vi "FPGA Resampling (60 Hz).vi"(0 "signal in":fxp<+/-,24,1>, 1 "number of channels":T3=7 items=["1"=1, "2"=2, "3"=3, "4"=4, "5"=5, "6"=6, "7"=7, "8"=8, "9"=9, "10"=10, "11"=11, "12"=12, "13"=13, "14"=14, "15"=15, "16"=16, "17"=17, "18"=18, "19"=19, "20"=20, "21"=21, "22"=22, "23"=23, "24"=24, "25"=25, "26"=26, "27"=27, "28"=28, "29"=29, "30"=30, "31"=31, "32"=32], 5 "timestamp [s]":fxp<+,64,32> format="%.42g", 7 "reference channel index (0)":u8, 9 "input valid? (T)":bool=TRUE, 12 "ready for output? (T)":bool=TRUE, 13 "samples per cycle (192)":u16=192) -> (4 "resampled data":T2, 6 "resampling info":T1={"nominal frequency"=enum."50 Hz", "resampling valid?"=FALSE, "samples per cycle"=192}, 10 "output valid?":bool, 15 "error":i32)   [LabVIEW 2014, in "NI_EP_Resample_FPGA.lvlib"]
doc: "Resamples even-time-spaced voltage and current signals into even-angle-spaced signals. The input signals must have a sample rate of 50 kHz. The output signals are synchronous with the line frequency with a constant number of samples per cycle. Use the Resampling for Power Quality VI if you want to perform resampling on the host computer. You must manually select the polymorphic instance to use.\n\nThis VI supports measuring single-bus single-line and single-bus multiple-line systems."
uses:
  <vilib>/addons/Electrical Power/PQ/Resampling/NI_EP_Resample_FPGA.lvlib
  <vilib>/addons/Electrical Power/PQ/Resampling/FPGA/subVIs/fpga_Typedef Fnom.ctl
  <vilib>/addons/Electrical Power/PQ/Resampling/FPGA/subVIs/fpga_Resampling Info.ctl
  <vilib>/addons/Electrical Power/PQ/Resampling/FPGA/subVIs/fpga_Resampled.ctl
  <vilib>/addons/Electrical Power/PQ/Resampling/FPGA/subVIs/fpga_NofCH (32ch).ctl
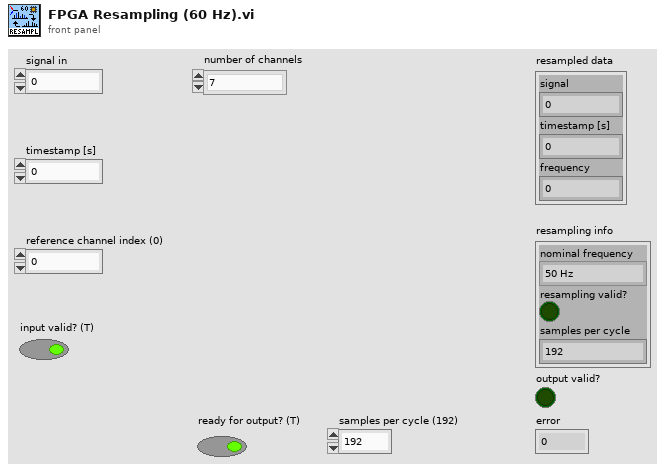
[diagram p1: front panel]
types:
  T1 = typedef "NI_EP_Resample_FPGA.lvlib/fpga_Resampling Info.ctl" = cluster{"nominal frequency":enum16{"50 Hz", "60 Hz"}, "resampling valid?":bool, "samples per cycle":u16}
  T2 = typedef "NI_EP_Resample_FPGA.lvlib/fpga_Resampled.ctl" = cluster{"signal":fxp<+/-,32,3>, "timestamp [s]":fxp<+,64,32>, "frequency":fxp<+,32,8>}
  T3 = typedef "NI_EP_Resample_FPGA.lvlib/fpga_NofCH (32ch).ctl" = u8
  T4 = typedef "NI_EP_Resample_FPGA.lvlib/fpga_Typedef Fnom.ctl" = u8
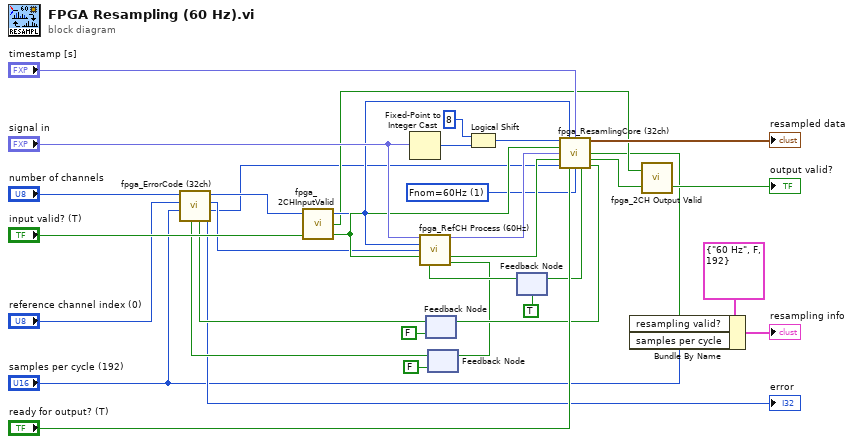
[diagram p0: block diagram]
diagram:
  w14 = T4 1 items=["Fnom=50Hz", "Fnom=60Hz"] ("Fnom")
  n1 = Fixed-Point to Integer Cast(1:"signal in") -> (0:w22:i32)
  n2 = feedback #1(FALSE) -> (w5:bool)
  n3 = feedback #2(FALSE) -> (w6:bool)
  n4 = call <vilib>:"fpga_ErrorCode (32ch).vi"("resampling FIFO time in"=w5, "Ref filter FIFO time in"=w6, "samples per cycle"="samples per cycle (192)", "reference channel index"="reference channel index (0)", "number of channels"="number of channels") -> ("error"=→"error":i32, "samples per cycle out"=w11:u16, "ref channel index out"=w12:u8, "number of CH out"=w13:u8)  [unwired: 3 in]
  n5 = call <vilib>:"fpga_2CHInputValid.vi"("input data valid"="input valid? (T)", "Channel number"=w13) -> ("input valid"=w24:bool, "1CH?"=w16:bool, "Channel number"=w17:u8)  [unwired: 1 in]
  n6 = Logical Shift(y=i8 8, x=w22) -> (x << y=w20:i32)
  n7 = feedback #3(TRUE ("Ready for reference input")) -> (w23:bool)
  n8 = call <vilib>:"fpga_RefCH Process (60Hz).vi"("data in <?24.1>"="signal in", "Channel number"=w17, "Reference index"=w12, "input data valid"=w24, "ready for output"=w23) -> ("Filtered Ref data <24,3>"=w19:fxp<+/-,24,3>, "output valid"=w18:bool, "Timed Out"=w7:bool)  [unwired: 8 in]
  n9 = feedback-in #2(w7) -> ()
  n10 = call <vilib>:"fpga_ResamlingCore (32ch).vi"("data in"=w20, "Channel number"=w17, "timestamp"="timestamp [s]", "input data valid"=w24, "reference in"=w19, "input reference valid"=w18, "interpolation factor"=w11, "Ready for output"="ready for output? (T)", "Fnom"=w14) -> ("Resample data and time"=→"resampled data":T2, "resampling valid"=w3:bool, "output valid"=w15:bool, "Ready for reference input"=w26:bool, "FIFO timeout?"=w9:bool)  [unwired: 2 in]
  n11 = feedback-in #1(w9) -> ()
  n12 = feedback-in #3(w26) -> ()
  n13 = Bundle By Name(cluster=T1 {"nominal frequency"=enum."60 Hz", "resampling valid?"=FALSE, "samples per cycle"=192} ("resampling info"), "resampling valid?"=w3, "samples per cycle"="samples per cycle (192)") -> (→"resampling info":T1)
  n14 = call <vilib>:"fpga_2CH Output Valid.vi"("output valid"=w15, "1CH?"=w16) -> ("output valid"=→"output valid?":bool)  [unwired: 1 in]
